vi "readFromXML.vi"(8 "error in (no error)":errorcluster, 10 "XML in":string, 11 "ScienceTargetOffset in":refnum<class "ScienceTargetOffset.lvclass">) -> (0 "error out":errorcluster, 3 "ScienceTargetOffset out":refnum<class "ScienceTargetOffset.lvclass">)   [LabVIEW 2022 SP3, in "TCSDataDefinitions.lvlib" / "TCSCommand.lvlib" / "OffsetCommands.lvlib" / "ScienceTargetOffset.lvclass"]
uses:
  ScienceTargetOffset.lvclass
  Offset/Offset.lvclass
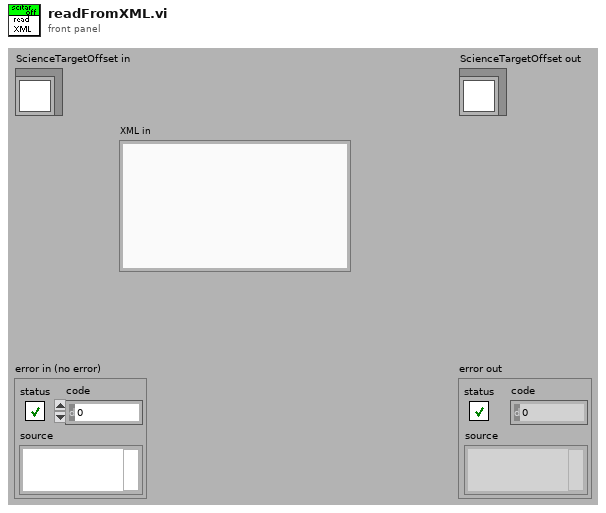
[diagram p1: front panel]
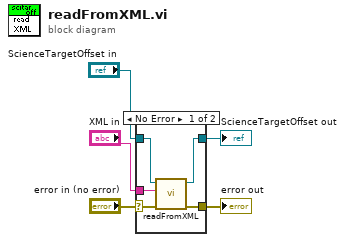
[diagram p0: block diagram]
diagram:
  n1 = case shown="No Error" "error in (no error)" {
    selector: "error in (no error)" -> [w9 w12]
    tunnel: [w8 w12] -> w4
    tunnel: [w6 w11] -> w2
    tunnel: "ScienceTargetOffset in" -> [w7 w11]
    tunnel: "XML in" -> [w10 _]
    frame No Error {
      n2 = call-parent "readFromXML.vi"("error in (no error)"=w9, "XML in"=w10, "Offset in"=w7) -> ("error out"=w8:errorcluster, "Offset out"=w6:refnum<class "ScienceTargetOffset.lvclass">)  [unwired: 7 out]
    }
    frame Error {
    }
  }
  "error out" <- w4
  "ScienceTargetOffset out" <- w2
